vi "U6 easy Stream Burst.vi"(8 "error in":errorcluster, 9 "# of Scans":dbl=1000.0 format="%.3f", 10 "Scan Rate (Hz)":dbl=1000.0 format="%.3f", 11 "Scan List (+)":u8[](array[numeric])=[0, 1, 2, 3]) -> (0 "error out":errorcluster, 2 "Data":dbl[][](array[numeric]) format="%.3f")   [LabVIEW 2021]
panel:
  out "Waveform Graph":dbl[][](graph)
  out "Error Message":string
  # "This example streams from the first found USB U6.  It does not read in a loop, but rather just does a single read with the desired number of\nscans.  Similar to Burst mode on the U12."
  # "The + scan list is the positive\nchannels.  This example will just\nuse 199 for negative channels\nmeaning single-ended.\n\nTo remove an element, right-click\non it, select Data Operations =>\nRemove Element.\n\nTo empty an array, right-click\nnear the edge, select Data\nOperations => Empty Array.\n\nOther useful operations:  From the\nOperate menu are \"Make Current\nValues Default\" and \"Reinitialize\nTo Default\"."
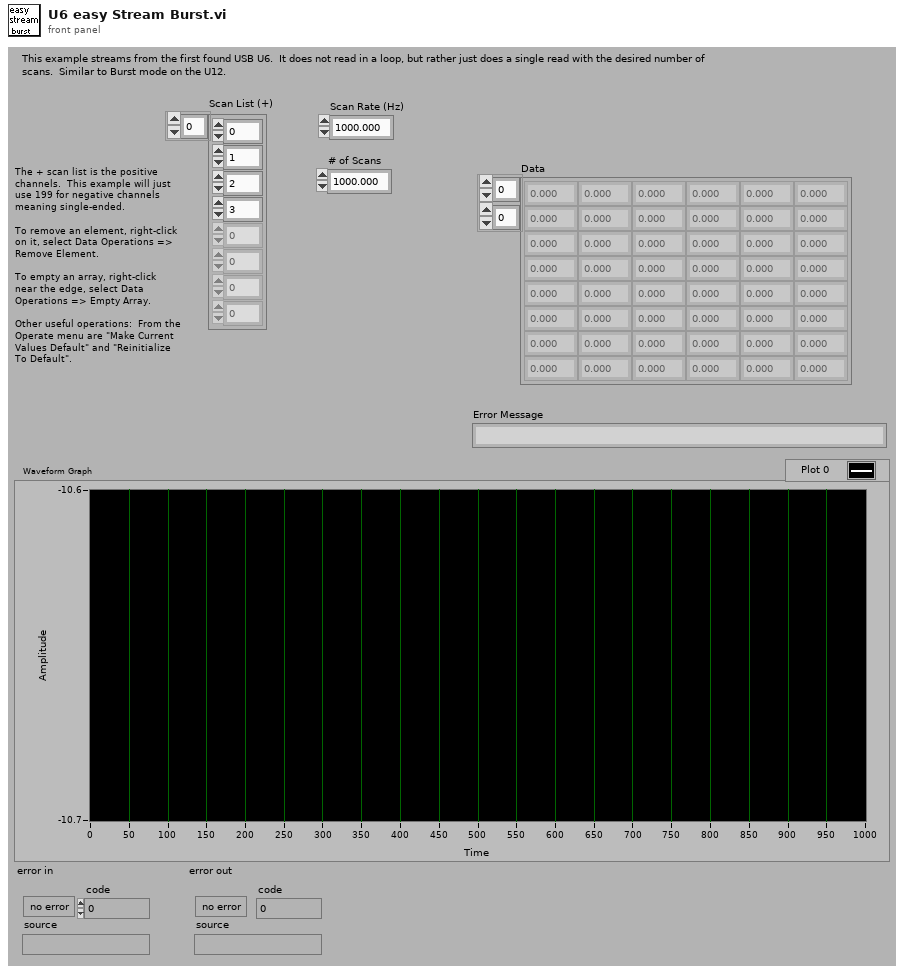
[diagram p1: front panel]
types:
  T1 = cluster{"PC buffer size (seconds)":dbl, "Resolution Index":u8, "StreamSettlingFactor":i32, "Binary":bool}
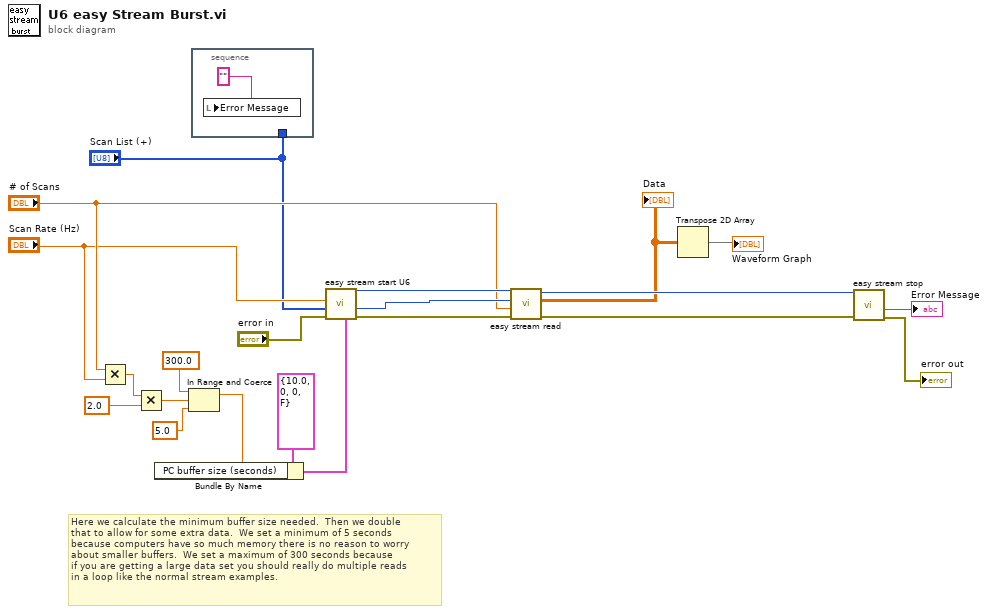
[diagram p0: block diagram]
diagram:
  # "Here we calculate the minimum buffer size needed.  Then we double\nthat to allow for some extra data.  We set a minimum of 5 seconds\nbecause computers have so much memory there is no reason to worry\nabout smaller buffers.  We set a maximum of 300 seconds because\nif you are getting a large data set you should really do multiple reads\nin a loop like the normal stream examples."
  n1 = Multiply(x="# of Scans", y="Scan Rate (Hz)") -> (x*y=w11:dbl)
  n2 = Multiply(x=w11, y=2.0) -> (x*y=w6:dbl)
  n3 = In Range and Coerce(upper limit=300.0, x=w6, lower limit=5.0) -> (coerced(x)=w4:dbl)  [unwired: 1 out]
  n4 = Bundle By Name(cluster=T1 {"PC buffer size (seconds)"=10.0, "Resolution Index"=0, "StreamSettlingFactor"=0, "Binary"=FALSE} ("Advanced"), "PC buffer size (seconds)"=w4) -> (w9:T1)
  n5 = stacked-sequence {
    tunnel: "Scan List (+)" -> [_]
    frame #0 {
      n6 = local write "Error Message"("" ("Error Message")) -> ()
    }
  }
  n7 = call "easy stream start U6.vi"("Advanced"=w9, "error in"="error in", "Scan List (+)"="Scan List (+)", "Scan Rate (Hz)"="Scan Rate (Hz)") -> ("error out"=w17:errorcluster, "# Channels"=w21:i32, "Handle Out"=w20:i32)  [unwired: 4 in, 1 out]
  n8 = call "easy stream read.vi"("error in"=w17, "Scans To Read"="# of Scans", "# Channels In Stream"=w21, "Handle In"=w20) -> ("error out"=w14:errorcluster, "Data"=w15:dbl[][], "Handle Out"=w19:i32)  [unwired: 4 in, 1 out]
  "Data" <- w15
  n9 = Transpose 2D Array(2D array=w15) -> (transposed array=→"Waveform Graph":dbl[][])
  n10 = call "easy stream stop.vi"("error in"=w14, "Handle In"=w19) -> ("error out"=→"error out":errorcluster, "Error Message"=→"Error Message":string)  [unwired: 7 in, 1 out]
